vi "close.vi"(8 "error in (no error)":errorcluster, 11 "NetworkWinX32 in":refnum<class "NetworkWinX32.lvclass">) -> (0 "error out":errorcluster)   [LabVIEW 2011, in "Hardware.lvlib" / "HWControllers.lvlib" / "NetworkWinX32.lvclass"]
uses:
  NetworkWinX32.lvclass
  NetworkWinX32.lvclass/NetworkWinX32.ctl
  Channels/Camera/WinX32_SA/WinX32Camera.lvclass
  NetworkCamera.lvclass
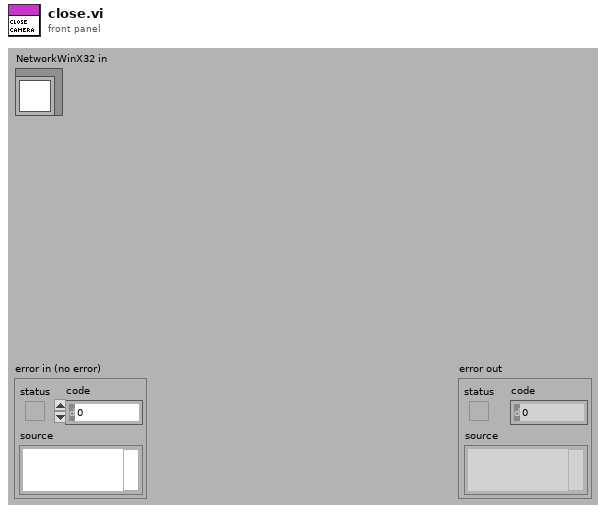
[diagram p1: front panel]
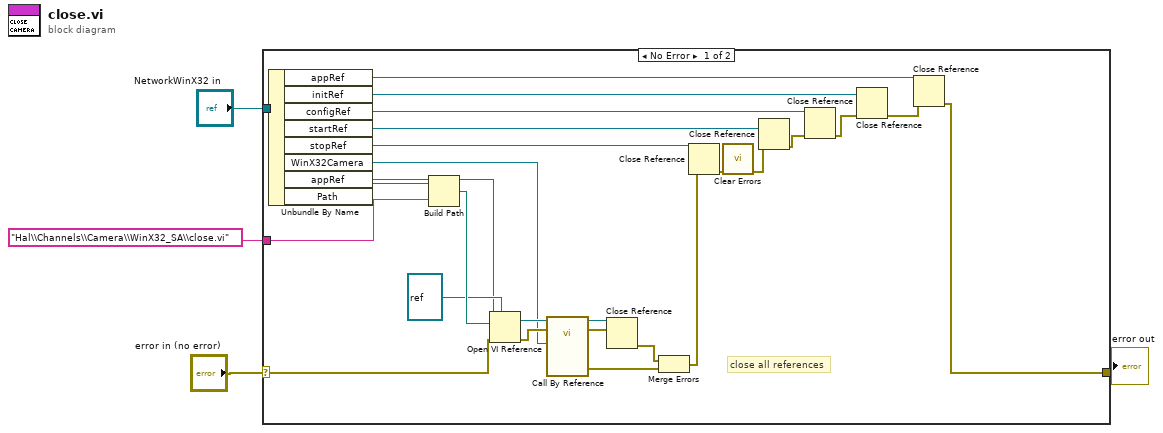
[diagram p0: block diagram]
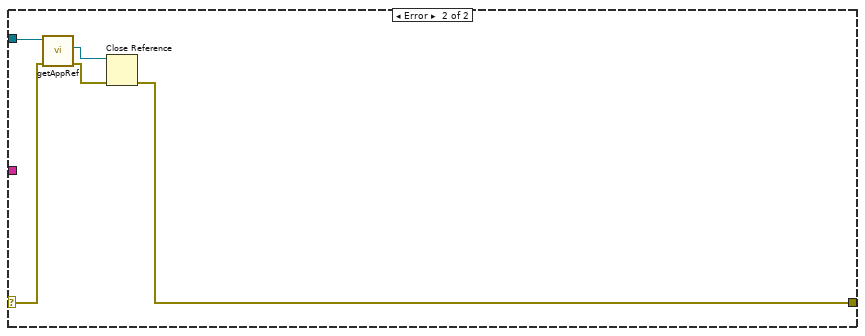
[diagram p2: hidden frame]
diagram:
  n1 = case shown="No Error" "error in (no error)" {
    selector: "error in (no error)" -> [w17 w34]
    tunnel: [w6 w31] -> w1
    tunnel: "NetworkWinX32 in" -> [w27 w35]
    tunnel: "Hal\\Channels\\Camera\\WinX32_SA\\close.vi" ("viPath") -> [w29 _]
    frame No Error {
      # "close all references"
      n2 = Unbundle By Name(w27) -> ("appRef"=w8:refnum<vi>, "initRef"=w10:refnum<vi>, "configRef"=w12:refnum<vi>, "startRef"=w14:refnum<vi>, "stopRef"=w15:refnum<vi>, "WinX32Camera"=w16:refnum<class "WinX32Camera.lvclass">, "appRef"=w18:refnum<vi>, "Path"=w26:path)
      n3 = Build Path(base path=w26, name or relative path=w29) -> (appended path=w30:path)
      n4 = Open VI Reference(type specifier VI Refnum (for type only)=refnum<vi> refnum, application reference (local)=w18, vi path=w30, error in (no error)=w17) -> (vi reference=w23:refnum<vi>, error out=w24:errorcluster)  [unwired: 2 in]
      n5 = call-by-ref "?"(reference=w23, error in=w24, "WinX32Camera in"=w16) -> (reference out=w21:refnum<vi>, error out=w22:errorcluster, 0:"error out"=w19:errorcluster)  [unwired: 9 in, 1 out]
      n6 = Close Reference(reference=w21, error in (no error)=w22) -> (error out=w20:errorcluster)
      n7 = Merge Errors(w20, w19) -> (w28:errorcluster)
      n8 = Close Reference(reference=w15, error in (no error)=w28) -> (error out=w13:errorcluster)
      n9 = call <vilib>:"Clear Errors.vi"("error in (no error)"=w13) -> ("error out"=w5:errorcluster)  [unwired: 6 in]
      n10 = Close Reference(reference=w14, error in (no error)=w5) -> (error out=w11:errorcluster)
      n11 = Close Reference(reference=w12, error in (no error)=w11) -> (error out=w9:errorcluster)
      n12 = Close Reference(reference=w10, error in (no error)=w9) -> (error out=w7:errorcluster)
      n13 = Close Reference(reference=w8, error in (no error)=w7) -> (error out=w6:errorcluster)
    }
    frame Error {
      n14 = call "getAppRef.vi"("error in (no error)"=w34, "NetworkCamera in"=w35) -> ("error out"=w32:errorcluster, "appRef"=w33:refnum<vi>)  [unwired: 7 in, 1 out]
      n15 = Close Reference(reference=w33, error in (no error)=w32) -> (error out=w31:errorcluster)
    }
  }
  "error out" <- w1
